vi "2-11.vi"() -> ()   [LabVIEW 2022 SP3]
panel:
  out "字符串":string
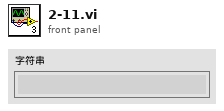
[diagram p1: front panel]
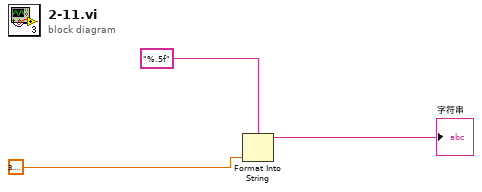
[diagram p0: block diagram]
diagram:
  n1 = Format Into String(format string="%.5f", 3.141592653589793) -> (resulting string=→"字符串":string)  [unwired: 2 in, 1 out]
